vi "test Compute VS Channel Handle Indices.vi"(8 "error in (no error)":errorcluster, 11 "TestCase in":refnum<class "Engine.lvclass">) -> (0 "error out":errorcluster, 3 "TestCase out":refnum<class "Engine.lvclass">)   [LabVIEW 2020, in "Engine.lvclass"]
uses:
  Engine.lvclass
  Shared/Direction.ctl
  <vilib>/NI VeriStand/Custom Device API/Custom Device Item Ref.ctl
  Engine/Custom Device/Compiled Message.ctl
  Shared/Parameter Definition.ctl
  <vilib>/addons/_JKI Toolkits/VI Tester/TestCase.llb/TestCase.lvclass
  Engine/Implementation/Execution Unit/Execution Unit.lvclass
  <vilib>/NI VeriStand/Custom Device API/Custom Device API.lvlib
  Engine/Custom Device/Custom Device.lvlib
  C:/Program Files (x86)/National Instruments/LabVIEW 2020/vi.lib/addons/_JKI Toolkits/VI Tester/TestCase.llb/TestCase.lvclass
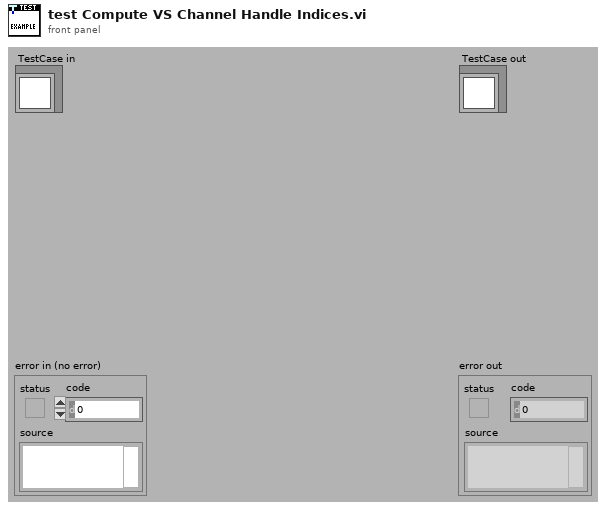
[diagram p1: front panel]
types:
  T1 = typedef "Direction.ctl" = enum16{"Rx", "Tx"}
  T2 = typedef "AIM MIL-STD-1553 Engine.lvlib/Custom Device.lvlib/Compiled Message.ctl" = cluster{"Message Section Handle":T3, "First Parameter Index":i32, "Parameter Channel Handles":T3[], "Direction":T1, "Parameters":T4[], "Receiving RT Address":u8, "Receiving RT Sub-address":u8, "Transmitting RT Address":u8, "Transmitting RT Sub-address":u8, "Word Count":u8, "Buffer Type":enum16{"unknown", "BC Message Buffer", "RT Message Buffer"}, "Buffer ID":u16, "Terminal Type":enum16{"Bus Controller", "Remote Terminal"}, "Timestamp Enabled":bool, "Timestamp Channel Handle":T3}
  T3 = typedef "Custom Device API.lvlib/Custom Device Item Ref.ctl" = u64
  T4 = typedef "Parameter Definition.ctl" = cluster{"start index":i32, "size (bits)":i32, "encoding":enum16{"BNR", "BCD", "Discrete"}, "signed":bool, "multiplier":dbl, "offset":dbl}
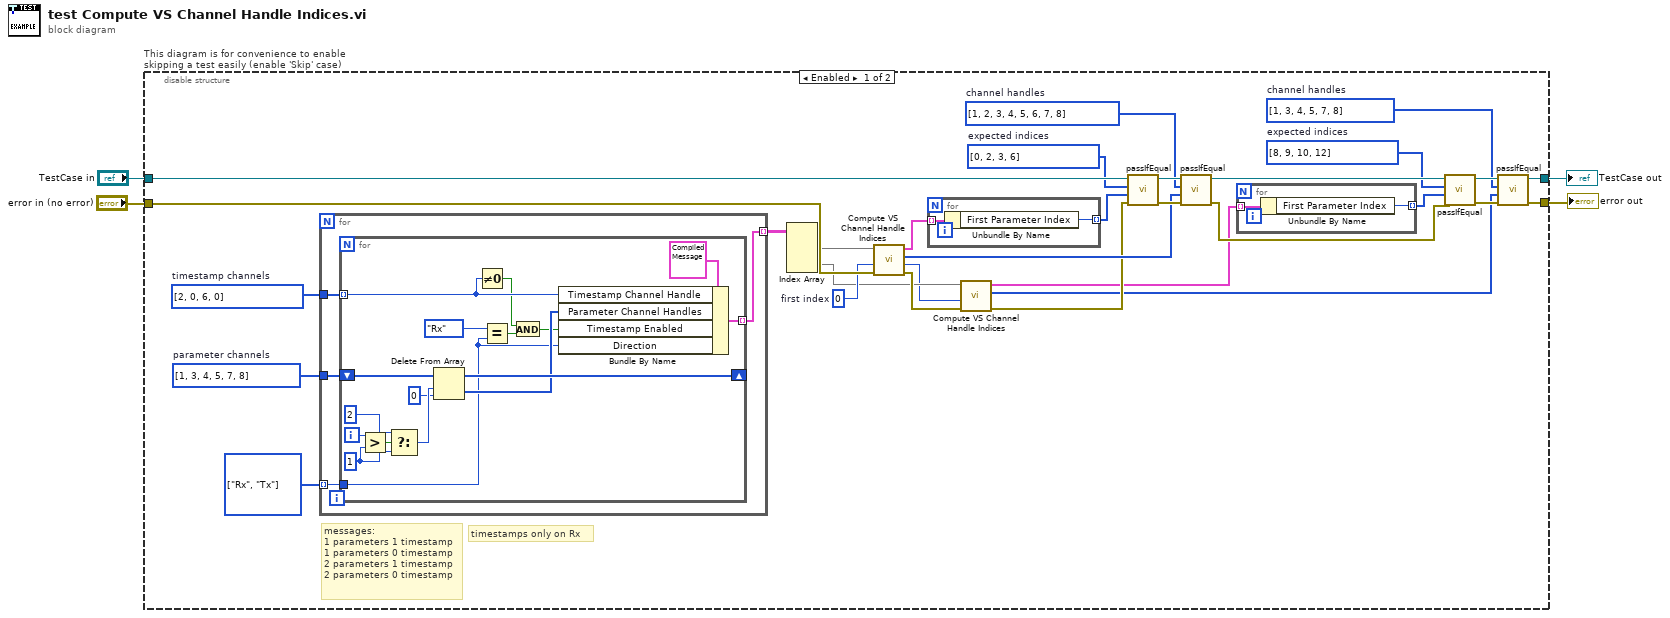
[diagram p0: block diagram]
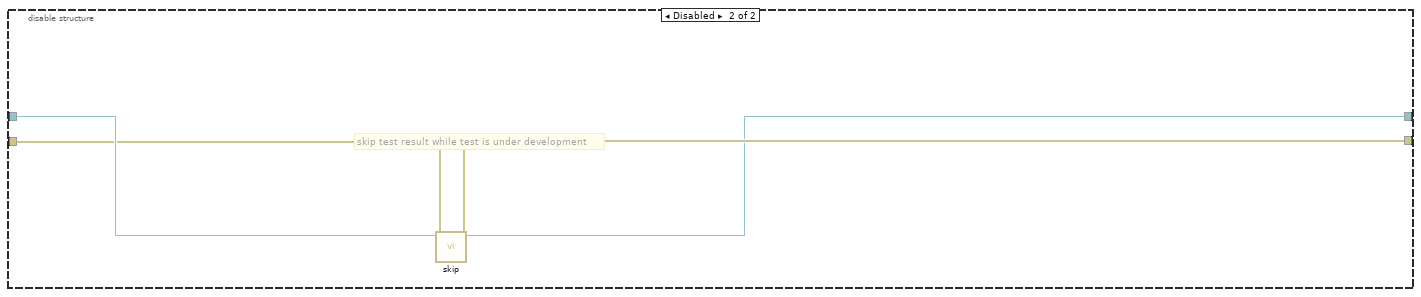
[diagram p2: hidden frame]
diagram:
  n1 = disable-structure "This diagram is for convenience to enable skipping a test easily (enable 'Skip' case)" shown="Enabled" {
    disable-tunnel: "TestCase in" -> [w32 w63]
    disable-tunnel: [w10 w61] -> w1
    disable-tunnel: [w9 w62] -> w3
    disable-tunnel: "error in (no error)" -> [w33 w60]
    frame Enabled {
      w5 = T3[] [1, 3, 4, 5, 7, 8]  # channel handles
      w6 = i32[] [8, 9, 10, 12]  # expected indices
      w23 = T3[] [1, 2, 3, 4, 5, 6, 7, 8]  # channel handles
      w28 = i32[] [0, 2, 3, 6]  # expected indices
      w29 = 0  # first index
      w30 = i32[] [1, 3, 4, 5, 7, 8]  # parameter channels
      w31 = T3[] [2, 0, 6, 0]  # timestamp channels
      w34 = T1[] [enum."Rx", enum."Tx"] items=["Rx", "Tx"] ("Direction")
      # "timestamps only on Rx"
      # "messages:\n1 parameters 1 timestamp\n1 parameters 0 timestamp\n2 parameters 1 timestamp\n2 parameters 0 timestamp"
      n2 = for {
        tunnel: w34 -> [w38] mode=indexing
        tunnel: [w37] -> w21 mode=indexing
        tunnel: w31 -> [w36]
        tunnel: w30 -> [w35]
        n3 = for {
          tunnel: w38 -> [w40]
          tunnel: [w54] -> w37 mode=indexing
          tunnel: w36 -> [w53] mode=indexing
          shift-right: [w47] -> _
          shift-left: w35 -> [w48]
          i -> [w52]
          w50 = 1 ("y")
          n4 = Greater?(x=w52, y=w50) -> (0:w51:bool)
          n5 = Select(t=2, s=w51, f=w50) -> (s? t:f=w46:i32)
          n6 = Delete From Array(array=w48, length=w46, index=0) -> (deleted portion=w45:i32[], array with subset deleted=w47:i32[])
          n7 = Not Equal To 0?(x=w53) -> (x != 0?=w43:bool)
          n8 = Equal?(x=Direction."Rx", y=w40) -> (x = y?=w41:bool)
          n9 = And(x=w43, y=w41) -> (x .and. y?=w42:bool)
          n10 = Bundle By Name(cluster=T2 {"Message Section Handle"=18446744073709551615, "First Parameter Index"=0, "Parameter Channel Handles"=[], "Direction"=enum."Rx", "Parameters"=[], "Receiving RT Address"=0, "Receiving RT Sub-address"=0, "Transmitting RT Address"=0, "Transmitting RT Sub-address"=0, "Word Count"=0, "Buffer Type"=enum."unknown", "Buffer ID"=0, "Terminal Type"=enum."Bus Controller", "Timestamp Enabled"=FALSE, "Timestamp Channel Handle"=0} ("messages and subaddresses"), "Timestamp Channel Handle"=w53, "Parameter Channel Handles"=w45, "Timestamp Enabled"=w42, "Direction"=w40) -> (w54:T2)
        }
      }
      n11 = Index Array(array=w21) -> (element #1=w20:T2[], element #2=w17:T2[])  [unwired: 4 in]
      n12 = call "Compute VS Channel Handle Indices.vi"("error in (no error)"=w33, "next index"=w29, "messages and subaddresses"=w20) -> ("error out"=w19:errorcluster, "next index out"=w16:i32, "channel handles"=w22:T3[], "messages and subaddresses out"=w27:T2[])  [unwired: 5 in]
      n13 = for {
        tunnel: w27 -> [w59] mode=indexing
        tunnel: [w58] -> w24 mode=indexing
        n14 = Unbundle By Name(w59) -> ("First Parameter Index"=w58:i32)
      }
      n15 = call "Compute VS Channel Handle Indices.vi"("error in (no error)"=w19, "next index"=w16, "messages and subaddresses"=w17) -> ("error out"=w18:errorcluster, "channel handles"=w7:T3[], "messages and subaddresses out"=w8:T2[])  [unwired: 5 in, 1 out]
      n16 = call-dynamic "passIfEqual.vi"("error in (no error)"=w18, "y"=w24, "x"=w28, "TestCase in"=w32) -> ("error out"=w25:errorcluster, "TestCase out"=w26:refnum<class "Engine.lvclass">)  [unwired: 6 in]
      n17 = call-dynamic "passIfEqual.vi"("error in (no error)"=w25, "y"=w22, "x"=w23, "TestCase in"=w26) -> ("error out"=w12:errorcluster, "TestCase out"=w11:refnum<class "Engine.lvclass">)  [unwired: 6 in]
      n18 = for {
        tunnel: w8 -> [w57] mode=indexing
        tunnel: [w56] -> w15 mode=indexing
        n19 = Unbundle By Name(w57) -> ("First Parameter Index"=w56:i32)
      }
      n20 = call-dynamic "passIfEqual.vi"("error in (no error)"=w12, "y"=w15, "x"=w6, "TestCase in"=w11) -> ("error out"=w14:errorcluster, "TestCase out"=w13:refnum<class "Engine.lvclass">)  [unwired: 6 in]
      n21 = call-dynamic "passIfEqual.vi"("error in (no error)"=w14, "y"=w7, "x"=w5, "TestCase in"=w13) -> ("error out"=w9:errorcluster, "TestCase out"=w10:refnum<class "Engine.lvclass">)  [unwired: 6 in]
    }
    frame Disabled {
      # "skip test result while test is under development"
      n22 = call <vilib>:"skip.vi"("error in (no error)"=w60, "TestCase in"=w63) -> ("error out"=w62:errorcluster, "TestCase out"=w61:refnum<class "Engine.lvclass">)  [unwired: 8 in]
    }
  }
  "error out" <- w3
  "TestCase out" <- w1
